vi "试剂容量设置UI.vi"() -> ()   [LabVIEW 2016]
panel:
  in  "试剂容量":T1 {"V 14" format="%.0f mL"; "V 13" format="%.0f mL"; "V 12" format="%.0f mL"; "V 11" format="%.0f mL"; "V 10" format="%.0f mL"; "V 9" format="%.0f mL"; "V 8" format="%.0f mL"; "V 7" format="%.0f mL"; "V 6" format="%.0f mL"; "V 5" format="%.0f mL"; "V 4" format="%.0f mL"; "V 3" format="%.0f mL"; "V 2" format="%.0f mL"; "V" format="%.0f mL"}
  in  "取消":bool
  in  "确认":bool
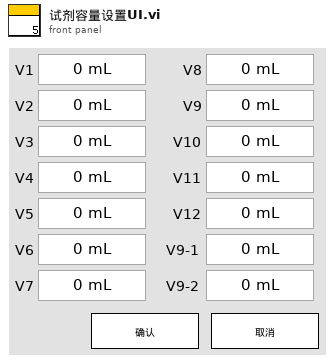
[diagram p1: front panel]
types:
  T1 = cluster{"V":u16, "V 2":u16, "V 3":u16, "V 4":u16, "V 5":u16, "V 6":u16, "V 7":u16, "V 8":u16, "V 9":u16, "V 10":u16, "V 11":u16, "V 12":u16, "V 13":u16, "V 14":u16}
  T2 = cluster{"时间标识":timestamp, "设备":string, "日志信息":string, "流程参数":string}
  T3 = cluster{"V1":sgl, "V2":sgl, "V3":sgl, "V4":sgl, "V5":sgl, "V6":sgl, "V7":sgl, "V8":sgl, "V9":sgl, "V10":sgl, "V11":sgl, "V12":sgl, "V9-1":sgl, "V9-2":sgl}
  T4 = cluster{"[0]":sgl, "[1]":sgl, "[2]":sgl, "[3]":sgl, "[4]":sgl, "[5]":sgl, "[6]":sgl, "[7]":sgl, "[8]":sgl, "[9]":sgl, "[10]":sgl, "[11]":sgl, "[12]":sgl, "[13]":sgl}
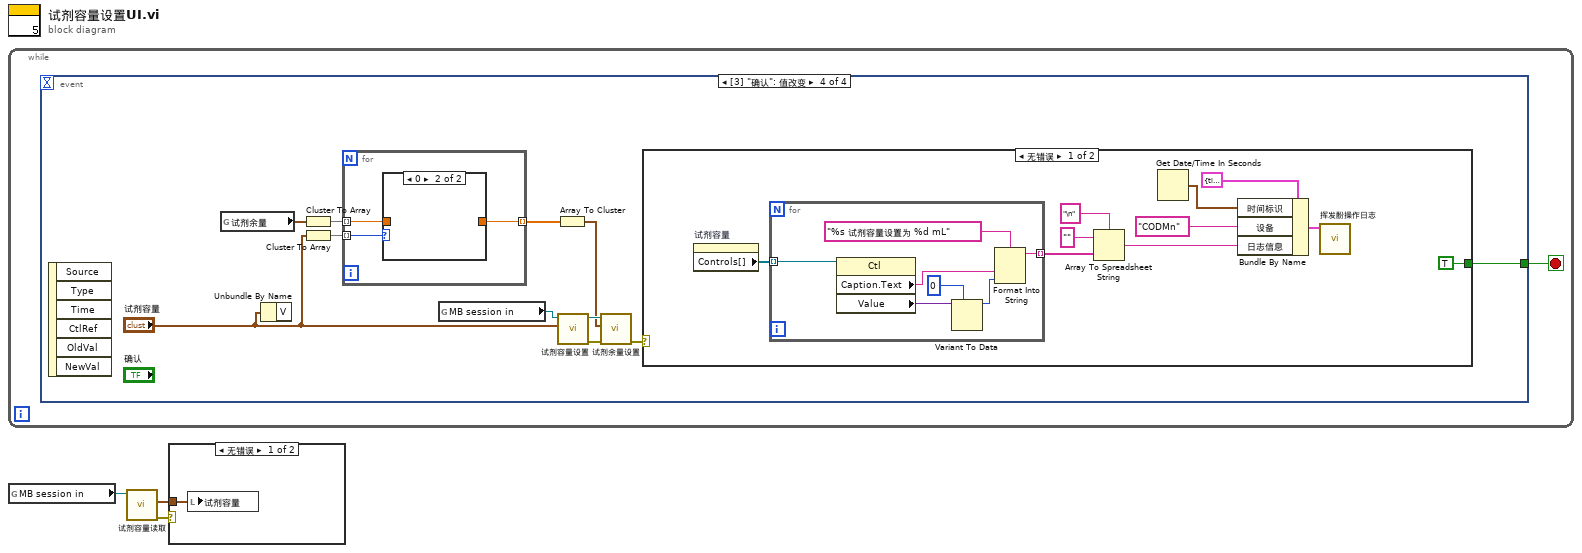
[diagram p0: block diagram]
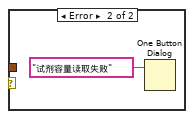
[diagram p2: hidden frame]
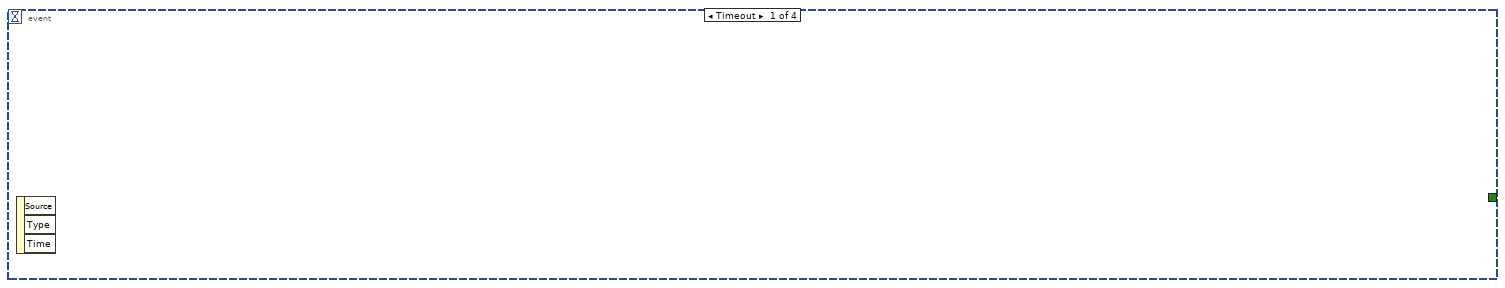
[diagram p3: hidden frame]
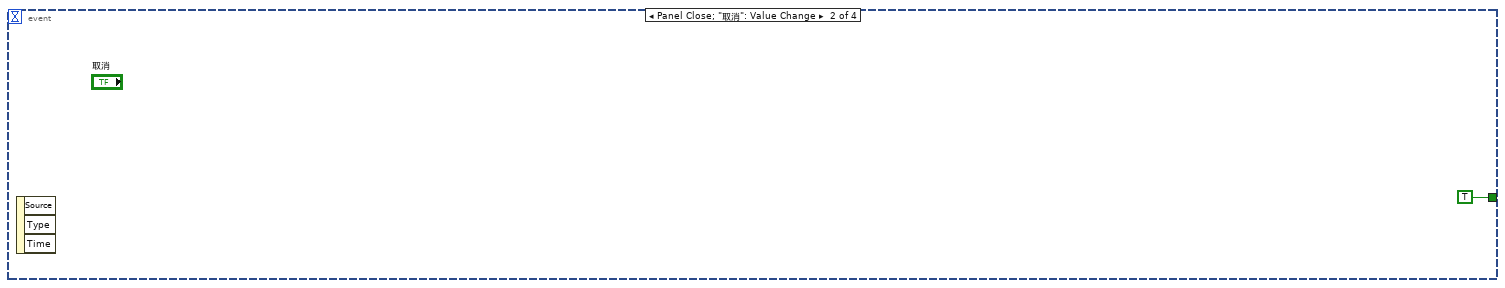
[diagram p4: hidden frame]
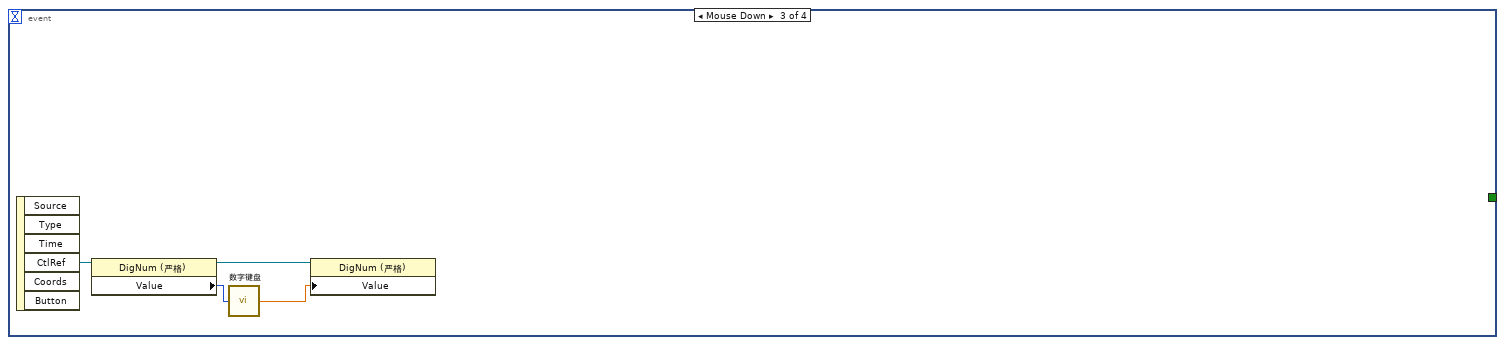
[diagram p5: hidden frame]
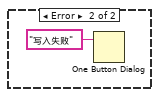
[diagram p7: hidden frame]
diagram:
  n1 = while {
    stop <- w4 stop-if-true
    n2 = event shown="[3] \"确认\": 值改变" {
      selector: _ -> [_ _ _ _]
      dyn-events: _ -> [_ _ _ _]
      timeout: _ -> [_ _ _ _]
      tunnel: [_ TRUE _ w20] -> w4
      event Timeout {
        n3 = event-data() -> ()  [unwired: 1 in, 3 out]
      }
      event Panel Close; "取消": Value Change {
        n4 = event-data() -> ()  [unwired: 1 in, 3 out]
      }
      event "试剂容量.V", "试剂容量.V 2", "试剂容量.V 3", "试剂容量.V 4", "试剂容量.V 5", "试剂容量.V 6", "试剂容量.V 7", "试剂容量.V 8", "试剂容量.V 9", "试剂容量.V 10", "试剂容量.V 11", "试剂容量.V 12", "试剂容量.V 13", "试剂容量.V 14": Mouse Down {
        n5 = event-data() -> ("CtlRef"=w9:refnum<vi>)  [unwired: 1 in, 5 out]
        n6 = property class="DigNum (严格)"(reference=w9) -> (reference out=w8:refnum<vi>, "Value"=w7:u16)  [unwired: 1 in, 1 out]
        n7 = call "数字键盘.vi"("OldNumber"=w7) -> ("NewNumber"=w6:dbl)
        n8 = property class="DigNum (严格)"(reference=w8, "Value"=w6) -> ()  [unwired: 1 in, 2 out]
      }
      event "确认": Value Change {
        n9 = event-data() -> ()  [unwired: 1 in, 6 out]
        n10 = global read "VAR挥发酚全局变量.vi" "试剂余量"() -> (w12:T3)
        n11 = Unbundle By Name("试剂容量") -> ()  [unwired: 1 out]
        n12 = Cluster To Array(cluster=w12) -> (array=w15:sgl[])
        n13 = Cluster To Array(cluster="试剂容量") -> (array=w16:u16[])
        n14 = for {
          tunnel: w16 -> [w23] mode=indexing
          tunnel: w15 -> [w21] mode=indexing
          tunnel: [w22] -> w14 mode=indexing
          n15 = case shown="0" w23 {
            tunnel: [w24 _] -> w22
            tunnel: w21 -> [w24 _]
            frame Default {
            }
            frame 0 {
            }
          }
        }
        n16 = global read "VAR挥发酚全局变量.vi" "MB session in"() -> (w18:refnum<class "MB_Master.lvclass">)
        n17 = Array To Cluster(array=w14) -> (cluster=w13:T4)
        n18 = call "试剂容量设置.vi"("试剂容量"="试剂容量", "MB session in"=w18) -> ("error out"=w11:errorcluster, "MB session out"=w17:refnum<class "MB_Master.lvclass">)  [unwired: 8 in]
        n19 = call "试剂余量设置.vi"("Error in"=w11, "试剂余量"=w13, "MB session in"=w17) -> ("error out"=w19:errorcluster)  [unwired: 7 in, 1 out]
        n20 = case shown="无错误" w19 {
          tunnel: [TRUE _] -> w20
          frame No Error {
            n21 = property on="试剂容量" class="Clust (严格)"() -> ("Controls[]"=w29:refnum<vi>[])  [unwired: 2 in, 2 out]
            n22 = for {
              tunnel: w29 -> [w41] mode=indexing
              tunnel: [w35] -> w31 mode=indexing
              n23 = property class="Ctl"(reference=w41) -> ("Caption.Text"=w36:string, "Value"=w38:variant)  [unwired: 1 in, 2 out]
              n24 = Variant To Data(type=u16 0 ("V"), Variant=w38) -> (data=w37:u16)  [unwired: 1 in, 1 out]
              n25 = Format Into String(format string="%s 试剂容量设置为 %d mL" ("格式字符串"), w36, w37) -> (resulting string=w35:string)  [unwired: 2 in, 1 out]
            }
            n26 = Array To Spreadsheet String(delimiter (Tab)="\n" ("分隔符(Tab)"), array=w31, 3:"" ("格式字符串")) -> (spreadsheet string=w33:string)
            n27 = Get Date/Time In Seconds() -> (seconds since 1Jan1904=w26:timestamp)
            n28 = Bundle By Name(cluster=T2 {"时间标识"=timestamp(0 s since 1904-01-01), "设备"="", "日志信息"="", "流程参数"=""} ("data in"), "时间标识"=w26, "设备"="CODMn", "日志信息"=w33) -> (w27:T2)
            n29 = call "挥发酚操作日志.vi"("data in"=w27) -> ()  [unwired: 11 in]
          }
          frame Error {
            n30 = One Button Dialog(message="写入失败" ("消息")) -> ()  [unwired: 1 in, 1 out]
          }
        }
      }
    }
  }
  n31 = global read "VAR挥发酚全局变量.vi" "MB session in"() -> (w3:refnum<class "MB_Master.lvclass">)
  n32 = call "试剂容量读取.vi"("MB session in"=w3) -> ("error out"=w2:errorcluster, "试剂容量"=w1:T3)  [unwired: 8 in, 1 out]
  n33 = case shown="无错误" w2 {
    tunnel: w1 -> [w43 _]
    frame No Error {
      n34 = local write "试剂容量"(w43) -> ()
    }
    frame Error {
      n35 = One Button Dialog(message="试剂容量读取失败" ("消息")) -> ()  [unwired: 1 in, 1 out]
    }
  }
